vi "IV_main.vi"() -> ()   [LabVIEW 2015, in "IV.lvlib"]
uses:
  IV.lvlib
panel:
  out "XY Graph 2":cluster{"X":dbl, "Y":dbl}[](graph)
  out "Error Out":errorcluster
  in  "Error In":errorcluster
  in  "Input parameters":T1={"Start Bias"=-3.0, "End Bias"=3.0, "Bias Step"=0.5, "High Resolution \nRegion"={"Start HR"=-0.5, "End HR"=0.5, "Bias Step HR"=0.1}}
  out "XY Graph":cluster{"Numeric":dbl, dbl}[](graph)
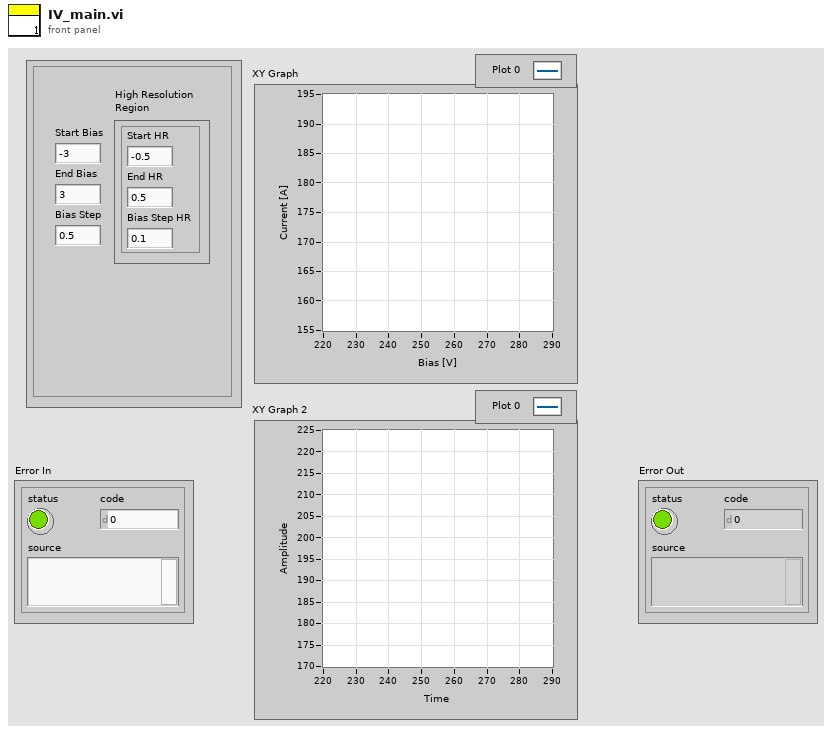
[diagram p1: front panel]
types:
  T1 = cluster{"Start Bias":dbl, "End Bias":dbl, "Bias Step":dbl, "High Resolution \nRegion":cluster{"Start HR":dbl, "End HR":dbl, "Bias Step HR":dbl}}
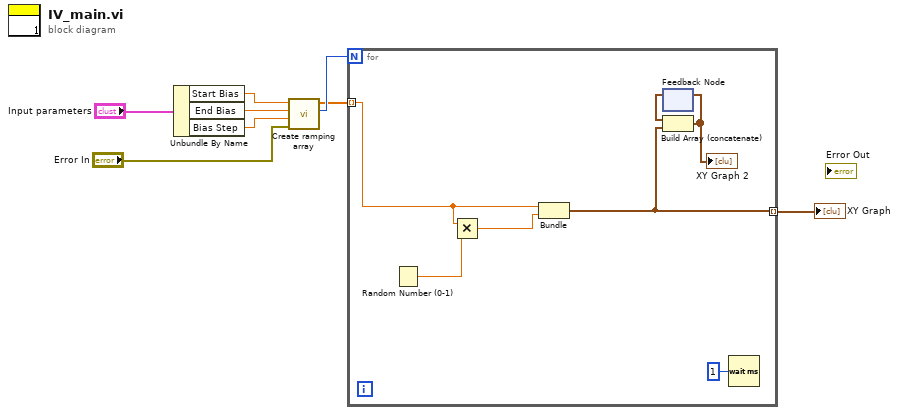
[diagram p0: block diagram]
diagram:
  n1 = Unbundle By Name("Input parameters") -> ("Start Bias"=w6:dbl, "End Bias"=w8:dbl, "Bias Step"=w7:dbl)
  n2 = call "Create ramping array.vi"("Error In"="Error In", "Delta"=w7, "End"=w8, "Start"=w6) -> ("Array length"=w4:i32, "Output Array (1D)"=w3:dbl[])  [unwired: 5 in, 1 out]
  n3 = for {
    N: w4 -> [_]
    tunnel: w3 -> [w12] mode=indexing
    tunnel: [w11] -> w2 mode=indexing
    n4 = Random Number (0-1)() -> (number: 0 to 1=w13:dbl)
    n5 = Multiply(x=w12, y=w13) -> (x*y=w14:dbl)
    n6 = Bundle("Numeric"=w12, w14) -> (w11:cluster{"Numeric":dbl, dbl})  [unwired: 1 in]
    n7 = feedback #1() -> (w10:cluster{"Numeric":dbl, dbl}[])  [unwired: 1 in]
    n8 = Build Array (concatenate)(w10, w11) -> (w9:cluster{"Numeric":dbl, dbl}[])
    "XY Graph 2" <- w9
    n9 = feedback-in #1(w9) -> ()
    n10 = Wait (ms)(milliseconds to wait=u32 1) -> ()  [unwired: 1 out]
  }
  "XY Graph" <- w2
